vi "Generate Lognormal Distribution.vi"(4 "type":u16(ring)=1 items=["Linear", "Logarithmic"], 5 "start":dbl=0.001 format="%#g", 6 "end":dbl=3.0 format="%0.2f", 7 "samples":i32=10000, 9 "Standard Dev":dbl=1.0, 10 "Geometric Mean":dbl=1.0, 11 "Number Concentration":dbl=20000.0) -> (3 "Distribution":cluster{dbl[], dbl[]}(graph))   [LabVIEW 2015]
doc: "Produce a lognormal distribution with mean diameter <B>Geometric Mean</B>, dispersion of <B>Standard Dev</B> and total number of particles of <B>Number Concentration</B>. The first bin will start at <B>start</B> and the final one will be bracketd by <B>end</B> with <B>samples</B>-1 bins spanning <B>end</B>-<B>start</B>. The y values will be determined based on the lognormal CDF while the x values are given as the geometric mean of the bin, or xm = sqrt(xu*xl)."
uses:
  <vilib>/Analysis/1siggen.llb/Ramp Pattern by Samples.vi
  <vilib>/gmath/NI_Gmath.lvlib
  <vilib>/Analysis/NI_AALBase.lvlib
panel:
  # "Spread of Diameters"
  # "Distribution Inputs"
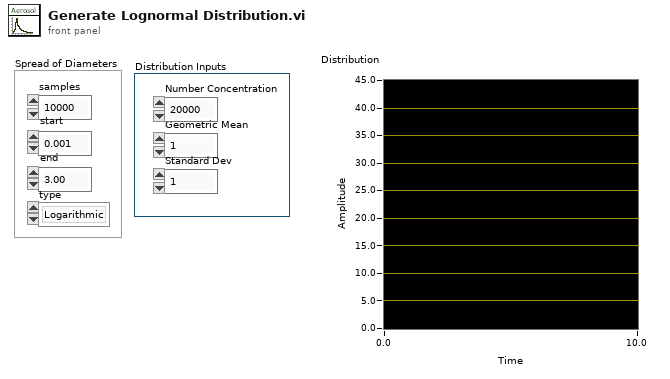
[diagram p1: front panel]
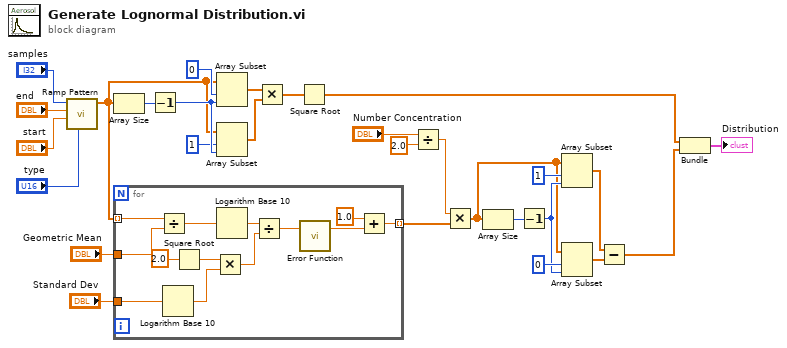
[diagram p0: block diagram]
diagram:
  n1 = call-poly <vilib>:"Ramp Pattern.vi"("type"="type", "start"="start", "end"="end", "samples"="samples") -> ("Ramp Pattern"=w2:dbl[])  [unwired: 6 in, 1 out]
  n2 = Array Size(array=w2) -> (size(s)=w10:i32)
  n3 = for {
    tunnel: w2 -> [w41] mode=indexing
    tunnel: "Geometric Mean" -> [w40]
    tunnel: "Standard Dev" -> [w38]
    tunnel: [w29] -> w20 mode=indexing
    n4 = Divide(x=w41, y=w40) -> (x/y=w35:dbl)
    n5 = Logarithm Base 10(1:w38) -> (0:w37:dbl)
    n6 = Square Root(x=2.0) -> (sqrt(x)=w36:dbl)
    n7 = Multiply(x=w36, y=w37) -> (x*y=w33:dbl)
    n8 = Logarithm Base 10(1:w35) -> (0:w34:dbl)
    n9 = Divide(x=w34, y=w33) -> (x/y=w31:dbl)
    n10 = call <vilib>:"Error Function.vi"("x"=w31) -> ("erf(x)"=w30:dbl)  [unwired: 2 in]
    n11 = Add(x=1.0, y=w30) -> (x+y=w29:dbl)
  }
  n12 = Decrement(x=w10) -> (x-1=w9:i32)
  n13 = Array Subset(array=w2, index=0, length=w9) -> (w6:dbl[])
  n14 = Array Subset(array=w2, index=1, length=w9) -> (w7:dbl[])
  n15 = Multiply(x=w6, y=w7) -> (x*y=w5:dbl[])
  n16 = Square Root(x=w5) -> (sqrt(x)=w4:dbl[])
  n17 = Divide(x="Number Concentration", y=2.0) -> (x/y=w19:dbl)
  n18 = Multiply(x=w19, y=w20) -> (x*y=w12:dbl[])
  n19 = Array Size(array=w12) -> (size(s)=w17:i32)
  n20 = Decrement(x=w17) -> (x-1=w16:i32)
  n21 = Array Subset(array=w12, index=1, length=w16) -> (w14:dbl[])
  n22 = Array Subset(array=w12, index=0, length=w16) -> (w13:dbl[])
  n23 = Subtract(x=w14, y=w13) -> (x-y=w1:dbl[])
  n24 = Bundle(w4, w1) -> (→"Distribution":cluster{dbl[], dbl[]})  [unwired: 1 in]
